vi "Execute.vi"(8 "error in (no error)":errorcluster, 9 "Workspace":T1, 10 "Control In":T2={"I-O.lvclass"=refnum, "Gantry"=refnum, "Dispenser"="COM1"}, 11 "Secure Syringe in":refnum<class "SecureRelease Syringe.lvclass">) -> (0 "error out":errorcluster, 2 "Control Out":T2={"I-O.lvclass"=refnum, "Gantry"=refnum, "Dispenser"="COM1"}, 3 "Secure Syringe out":refnum<class "SecureRelease Syringe.lvclass">)   [LabVIEW 2021, in "SecureRelease Syringe.lvclass"]
uses:
  SecureRelease Syringe.lvclass
  Controller/Controllers.ctl
  Controller/I-O/I-O.lvclass
  C:/Program Files (x86)/Aerotech/A3200/LabVIEW/2010/Bin/Aerotech.A3200.dll
  Program Files (x86)/Aerotech/A3200/LabVIEW/2010/Bin/Aerotech.A3200.dll
  Workspace/Workspace.ctl
  SecureRelease Syringe.lvclass/SecureRelease Syringe.ctl
  Controller/Motion/Motion.lvclass
  Dispense/Dispense.lvclass
  Controller/Motion/A3200/A3200.lvclass
  Controller/Dispenser/Dispenser.lvclass
  Controller/Controller.lvclass
  Workspace/Fixture.lvclass
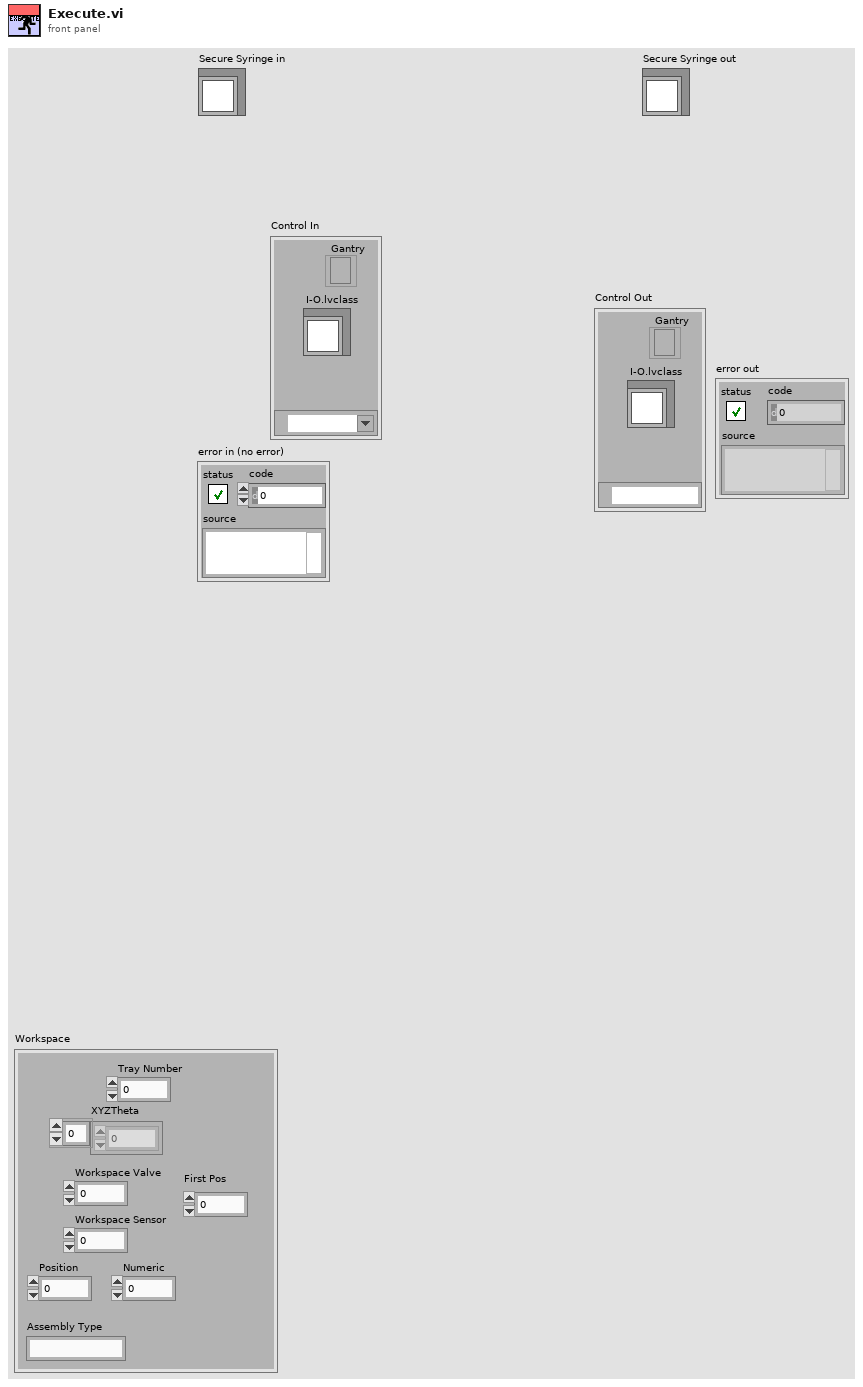
[diagram p1: front panel]
types:
  T1 = typedef "Fixture.lvclass/Workspace.ctl" = cluster{"XYZTheta":dbl[], "Workspace Valve":i32, "Workspace Sensor":i32, "Tray Number":i32, "Position":i32, "Assembly Type":string, "Numeric":dbl, "First Pos":i32}
  T2 = typedef "Controller.lvclass/Controllers.ctl" = cluster{"I-O.lvclass":refnum<class "I-O.lvclass">, "Gantry":refnum<k24>, "Dispenser":refnum<visa-resource-name>}
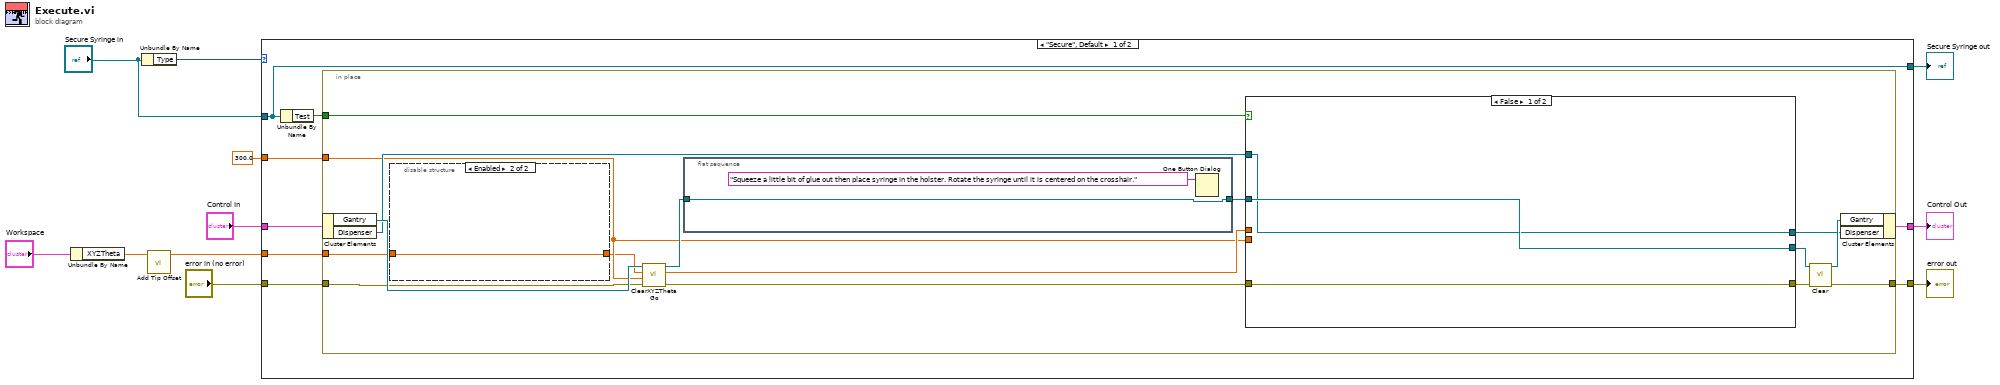
[diagram p0: block diagram]
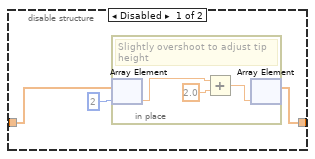
[diagram p2: hidden frame]
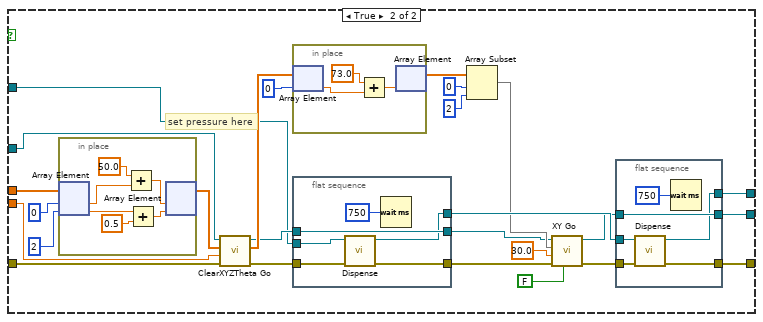
[diagram p3: hidden frame]
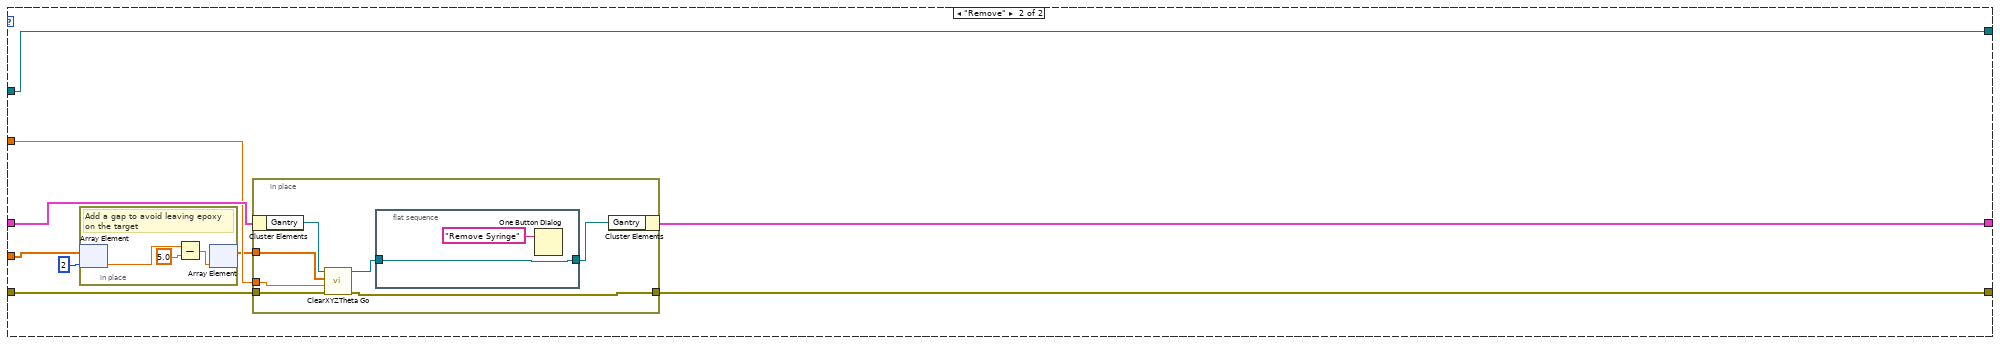
[diagram p4: hidden frame]
diagram:
  n1 = Unbundle By Name("Workspace") -> ("XYZTheta"=w4:dbl[])
  n2 = Unbundle By Name("Secure Syringe in") -> ("Type"=w6:enum16{"Secure", "Remove"})
  n3 = call "Add Tip Offset.vi"("XYZTheta"=w4) -> ("XYZTheta"=w3:dbl[])  [unwired: 10 in]
  n4 = case shown="\"Secure\", Default" w6 {
    tunnel: "Secure Syringe in" -> [w16 w101]
    tunnel: [w16 w101] -> w10
    tunnel: "Control In" -> [w19 w102]
    tunnel: [w18 w103] -> w8
    tunnel: 300.0 ("Speed") -> [w15 w100]
    tunnel: w3 -> [w14 w99]
    tunnel: "error in (no error)" -> [w13 w96]
    tunnel: [w12 w95] -> w1
    frame "Secure", Default {
      n5 = Unbundle By Name(w16) -> ("Test"=w17:bool)
      n6 = in-place {
        in-place-border: w17 -> [w29]
        in-place-border: w15 -> [w26]
        in-place-border: w14 -> [w25]
        in-place-border: w13 -> [w23]
        in-place-border: [w20] -> w12
        n7 = in-place-cluster #1(w19) -> ("Gantry"=w35:refnum<k24>, "Dispenser"=w28:refnum<visa-resource-name>)
        n8 = disable-structure shown="Enabled" {
          disable-tunnel: w25 -> [w38 w42]
          disable-tunnel: [w37 w42] -> w24
          frame Disabled {
            n9 = in-place {
              # "Slightly overshoot to adjust tip height"
              n10 = in-place-array #2(w38, 2) -> (w41:dbl)
              n11 = Add(x=w41, y=2.0) -> (x+y=w40:dbl)
              n12 = in-place-array #2(w40) -> (w37:dbl[])  [unwired: 1 out]
            }
          }
          frame Enabled {
          }
        }
        n13 = call "ClearXYZTheta Go.vi"("error in (no error)"=w23, "Speed"=w26, "XYZTheta In"=w24, "Gantry In"=w35) -> ("error out"=w22:errorcluster, "XYZTheta Out"=w30:dbl[], "Gantry Out"=w34:refnum<k24>)  [unwired: 5 in]
        n14 = flat-sequence {
          tunnel: [w93] -> w32
          tunnel: w34 -> [w93]
          frame #0 {
            n15 = One Button Dialog(message="Squeeze a little bit of glue out then place syringe in the holster. Rotate the syringe until it is centered on the crosshair.") -> ()  [unwired: 1 in, 1 out]
          }
        }
        n16 = case shown="False" w29 {
          tunnel: w32 -> [w45 w71]
          tunnel: [w45 w63] -> w31
          tunnel: w30 -> [_ w70]
          tunnel: w28 -> [w44 w53]
          tunnel: [w44 w61] -> w27
          tunnel: w26 -> [_ w51]
          tunnel: w22 -> [w43 w50]
          tunnel: [w43 w46] -> w21
          frame False {
          }
          frame True {
            # "set pressure here"
            n17 = in-place {
              n18 = in-place-array #3(w70, 0, 2) -> (w92:dbl, w90:dbl)
              n19 = Add(x=50.0, y=w92) -> (x+y=w87:dbl)
              n20 = Add(x=w90, y=0.5) -> (x+y=w88:dbl)
              n21 = in-place-array #3(w87, w88) -> (w67:dbl[])  [unwired: 2 out]
            }
            n22 = call "ClearXYZTheta Go.vi"("error in (no error)"=w50, "Speed"=w51, "XYZTheta In"=w67, "Gantry In"=w71) -> ("error out"=w49:errorcluster, "XYZTheta Out"=w66:dbl[], "Gantry Out"=w64:refnum<k24>)  [unwired: 5 in]
            n23 = in-place {
              n24 = in-place-array #4(w66, 0) -> (w86:dbl)
              n25 = Add(x=73.0, y=w86) -> (x+y=w84:dbl)
              n26 = in-place-array #4(w84) -> (w60:dbl[])  [unwired: 1 out]
            }
            n27 = flat-sequence {
              tunnel: [w83] -> w55
              tunnel: w64 -> [w83]
              tunnel: w53 -> [w80]
              tunnel: [w81] -> w62
              tunnel: w49 -> [w79]
              tunnel: [w78] -> w48
              frame #0 {
                n28 = call "Dispense.vi"("error in (no error)"=w79, "Dispenser In"=w80) -> ("error out"=w78:errorcluster, "Dispenser Out"=w81:refnum<visa-resource-name>)  [unwired: 8 in]
                n29 = Wait (ms)(milliseconds to wait=u32 750) -> ()  [unwired: 1 out]
              }
            }
            n30 = Array Subset(array=w60, index=0, length=2) -> (w57:dbl[])
            n31 = call "XY Go.vi"("return immediately"=FALSE, "error in (no error)"=w48, "Speed"=30.0, "XY In"=w57, "Gantry In"=w55) -> ("error out"=w47:errorcluster, "Gantry Out"=w54:refnum<k24>)  [unwired: 4 in, 1 out]
            n32 = flat-sequence {
              tunnel: [w77] -> w63
              tunnel: w54 -> [w77]
              tunnel: w62 -> [w74]
              tunnel: [w75] -> w61
              tunnel: w47 -> [w73]
              tunnel: [w72] -> w46
              frame #0 {
                n33 = call "Dispense.vi"("error in (no error)"=w73, "Dispenser In"=w74) -> ("error out"=w72:errorcluster, "Dispenser Out"=w75:refnum<visa-resource-name>)  [unwired: 8 in]
                n34 = Wait (ms)(milliseconds to wait=u32 750) -> ()  [unwired: 1 out]
              }
            }
          }
        }
        n35 = call "Clear.vi"("error in (no error)"=w21, "Gantry In"=w31) -> ("error out"=w20:errorcluster, "Gantry Out"=w33:refnum<k24>)  [unwired: 8 in]
        n36 = in-place-cluster #1("Gantry"=w33, "Dispenser"=w27) -> (w18:T2)
      }
    }
    frame "Remove" {
      n37 = in-place {
        # "Add a gap to avoid leaving epoxy on the target"
        n38 = in-place-array #5(w99, 2) -> (w105:dbl)
        n39 = Subtract(x=w105, y=5.0) -> (x-y=w106:dbl)
        n40 = in-place-array #5(w106) -> (w98:dbl[])  [unwired: 1 out]
      }
      n41 = in-place {
        in-place-border: w98 -> [w110]
        in-place-border: w100 -> [w109]
        in-place-border: w96 -> [w108]
        in-place-border: [w107] -> w95
        n42 = in-place-cluster #6(w102) -> ("Gantry"=w113:refnum<k24>)
        n43 = call "ClearXYZTheta Go.vi"("error in (no error)"=w108, "Speed"=w109, "XYZTheta In"=w110, "Gantry In"=w113) -> ("error out"=w107:errorcluster, "Gantry Out"=w112:refnum<k24>)  [unwired: 5 in, 1 out]
        n44 = flat-sequence {
          tunnel: w112 -> [w115]
          tunnel: [w115] -> w111
          frame #0 {
            n45 = One Button Dialog(message="Remove Syringe") -> ()  [unwired: 1 in, 1 out]
          }
        }
        n46 = in-place-cluster #6("Gantry"=w111) -> (w103:T2)
      }
    }
  }
  "error out" <- w1
  "Secure Syringe out" <- w10
  "Control Out" <- w8
